vi "Pre Launch Init.vi"(11 "EventHandlerTask in":refnum<class "EventHandlerTask.lvclass">) -> (0 "error out":errorcluster, 3 "EventHandlerTask out":refnum<class "EventHandlerTask.lvclass">)   [LabVIEW 2020, in "Volatus.lvlib" / "EventHandlerTask.lvclass"]
doc: "(<B>Filename</B>: Actor Framework.lvlib:Actor.lvclass:Pre Launch Init.vi)\n\nDefines behavior that occurs after the Launch Nested Actor method is invoked but before the actor's Actor Core method begins running.\n\nBy default, this method does nothing. A descendant class may override it to define behavior."
uses:
  EventHandlerTask.lvclass
  C:/Program Files (x86)/National Instruments/LabVIEW 2020/vi.lib/ActorFramework/Actor/Actor.lvclass
  C:/dev/lv20CE/relink/lv-volatus/Volatus/Task/Task.lvclass
  <vilib>/ActorFramework/Actor/Actor.lvclass/Actor.ctl
  <vilib>/ActorFramework/Message Enqueuer/Message Enqueuer.lvclass/Message Enqueuer.ctl
  Task/Task.lvclass/Task.ctl
  <vilib>/ActorFramework/Message Enqueuer/Init from Existing Queue.vi
  <vilib>/ActorFramework/Message Enqueuer/Message Enqueuer.lvclass
  Task/Task.lvclass
  EventHandlerTask.lvclass/EventHandlerTask.ctl
  Event API/EventAPI.lvclass
  <vilib>/ActorFramework/Actor/Actor.lvclass
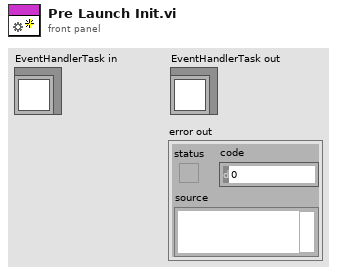
[diagram p1: front panel]
types:
  T1 = typedef "Volatus.lvlib/Core APIs.ctl" = cluster{"Volatus":refnum<class "VolatusAPI.lvclass">, "Event":refnum<class "EventAPI.lvclass">, "Telemetry":refnum<class "TelemetryAPI.lvclass">}
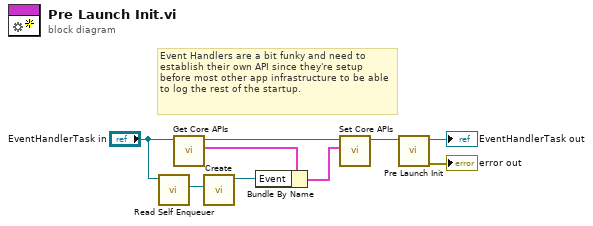
[diagram p0: block diagram]
diagram:
  # "Event Handlers are a bit funky and need to establish their own API since they're setup before most other app infrastructure to be able to log the rest of the startup."
  n1 = call <vilib>:"Read Self Enqueuer.vi"("Actor"="EventHandlerTask in") -> ("Self Enqueuer"=w9:refnum<class "Message Enqueuer.lvclass">)  [unwired: 10 in]
  n2 = call "Get Core APIs.vi"("Task in"="EventHandlerTask in") -> ("Core APIs"=w6:T1, "Task out"=w7:refnum<class "EventHandlerTask.lvclass">)  [unwired: 8 in, 1 out]
  n3 = call "Create.vi"("EnQr"=w9) -> ("Event API out"=w5:refnum<class "EventAPI.lvclass">)  [unwired: 9 in, 1 out]
  n4 = Bundle By Name(cluster=w6, "Event"=w5) -> (w3:T1)
  n5 = call "Set Core APIs.vi"("Core APIs"=w3, "Task in"=w7) -> ("Task out"=w4:refnum<class "EventHandlerTask.lvclass">)  [unwired: 8 in, 1 out]
  n6 = call-parent "Pre Launch Init.vi"("Task in"=w4) -> ("error out"=→"error out":errorcluster, "Task out"=→"EventHandlerTask out":refnum<class "EventHandlerTask.lvclass">)  [unwired: 9 in]
